vi "Start.vi"(8 "error in":errorcluster, 9 "timeout (-1)":i32=-1, 11 "Standard Engine in":refnum<class "Standard Engine Runtime.lvclass">) -> (0 "error out":errorcluster, 3 "Standard Engine out":refnum<class "Standard Engine Runtime.lvclass">)   [LabVIEW 2013, in "Standard Engine Runtime.lvclass"]
doc: "Sends a command for a paused but initialized engine to begin execution and enter the 'Running' state."
uses:
  Standard Engine Runtime.lvclass
  Commands.ctl
  <vilib>/NI/Module Execution Interface/Engine Runtime/Execution States.ctl
  Standard Engine Runtime.lvclass/Standard Engine Runtime.ctl
  <vilib>/NI/Module Execution Interface/Engine Runtime/Engine Runtime Interface.lvclass
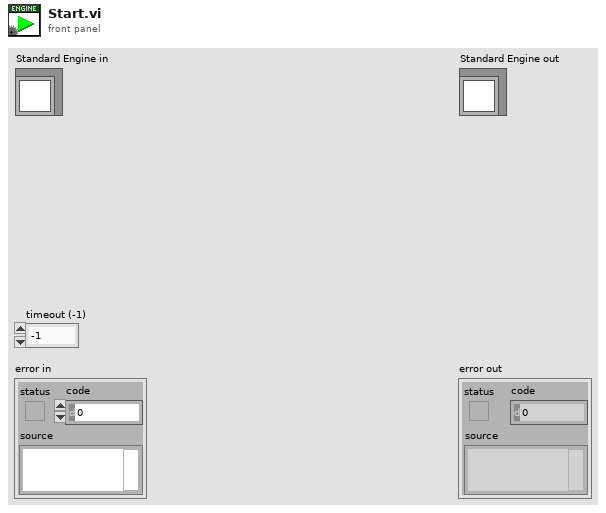
[diagram p1: front panel]
types:
  T1 = typedef "Engine Runtime Interface.lvclass/Execution States.ctl" = enum16{"Initializing", "Paused (Initialized)", "Running", "Set Safe Outputs", "Uninitializing", "Stopped (Uninitialized)", "Error (Uninitialized)", "Safe State (Uninitialized)", "Closed"}
  T2 = typedef "Standard Engine Runtime.lvclass/Commands.ctl" = enum16{"Initialize", "Start", "Pause", "Safe State", "Normal", "Stop", "Shutdown"}
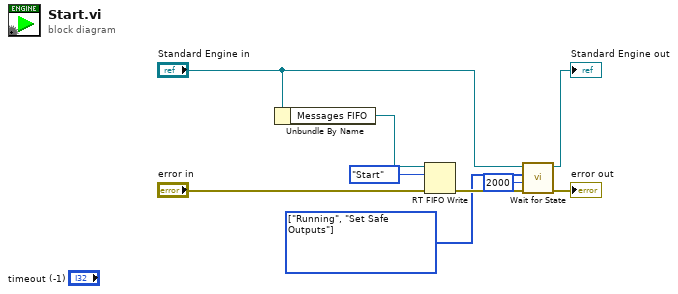
[diagram p0: block diagram]
diagram:
  w4 = T1[] [enum."Running", enum."Set Safe Outputs"] items=["Initializing", "Paused (Initialized)", "Running", "Set Safe Outputs", "Uninitializing", "Stopped (Uninitialized)", "Error (Uninitialized)", "Safe State (Uninitialized)", "Closed"] ("expected states")
  n1 = Unbundle By Name("Standard Engine in") -> ("Messages FIFO"=w9:refnum<k33>)
  n2 = RT FIFO Write(0:w9, 1:Commands."Start" ("element"), 3:"error in") -> (11:w6:errorcluster)  [unwired: 2 in, 3 out]
  n3 = call "Wait for State.vi"("error in"=w6, "timeout in ms"=2000, "expected states"=w4, "Standard Engine in"="Standard Engine in") -> ("error out"=→"error out":errorcluster, "Standard Engine out"=→"Standard Engine out":refnum<class "Standard Engine Runtime.lvclass">)  [unwired: 6 in]
